vi "N-216 Test Panel - DLL.vi"() -> ()   [LabVIEW 2016]
uses:
  PI GCS2 DLL/PI_GCS2_DLL_x64.dll
panel:
  in  "Num of Axes":i32=1
  out "Axes Names":string
  in  "Query All Connected":bool
  out "MVR Success":u8
  in  "Move Relative":dbl
  out "Set VEL Success":u8
  in  "Set Velocity (µm/s)":dbl
  out "Velocities":dbl[](array[numeric])
  in  "Get Velocity (um/sec)":bool
  out "Halt Cmd Success":u8
  in  "Halt":bool
  out "ONT? Success":u8
  out "ONT?":u8[](array[numeric])
  in  "Check On Target":bool
  out "MOV Cmd Success":u8
  in  "Move to Position (µm)":dbl
  out "Referencing":bool
  out "Reference Position":dbl[](array[numeric])
  in  "Perform REF":bool
  out "FRF?":u8[](array[numeric])
  out "FRF Success":u8
  in  "Check REF":bool
  out "SVO Return":u8
  in  "SVO":bool
  in  "Axis":string="1"
  in  "All Axis":bool=TRUE
  in  "Get SVO State":bool
  in  "Get Position":bool
  in  "Quit":bool
  out "Error Code":i32
  out "Servo States":u8[](array[numeric])
  out "Positions":dbl[](array[numeric])
  out "Device ID":i32
  out "PI USB Devices":string
  out "Number Connected":i32
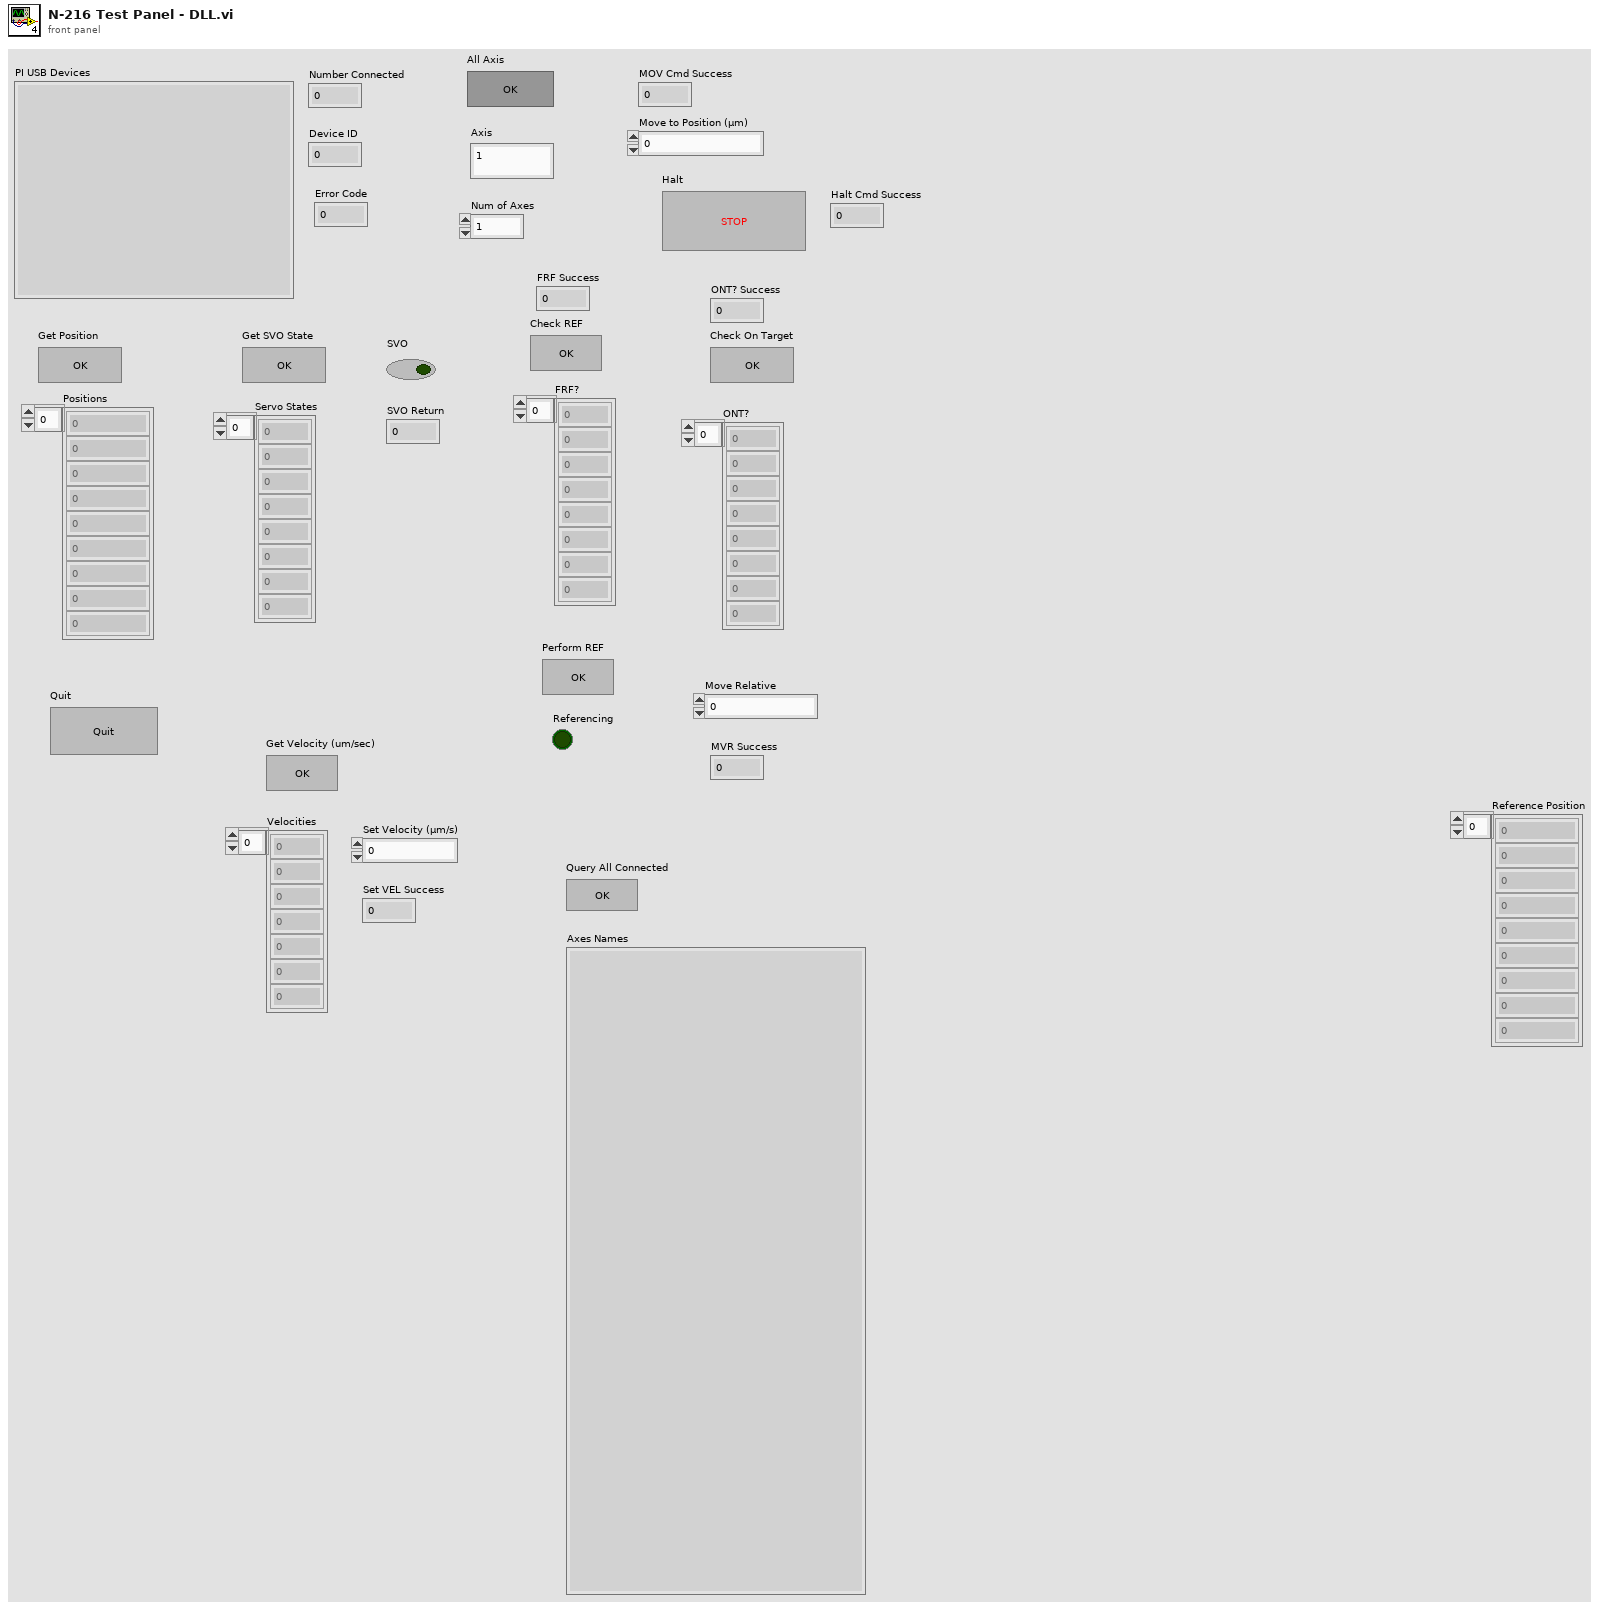
[diagram p1: front panel]
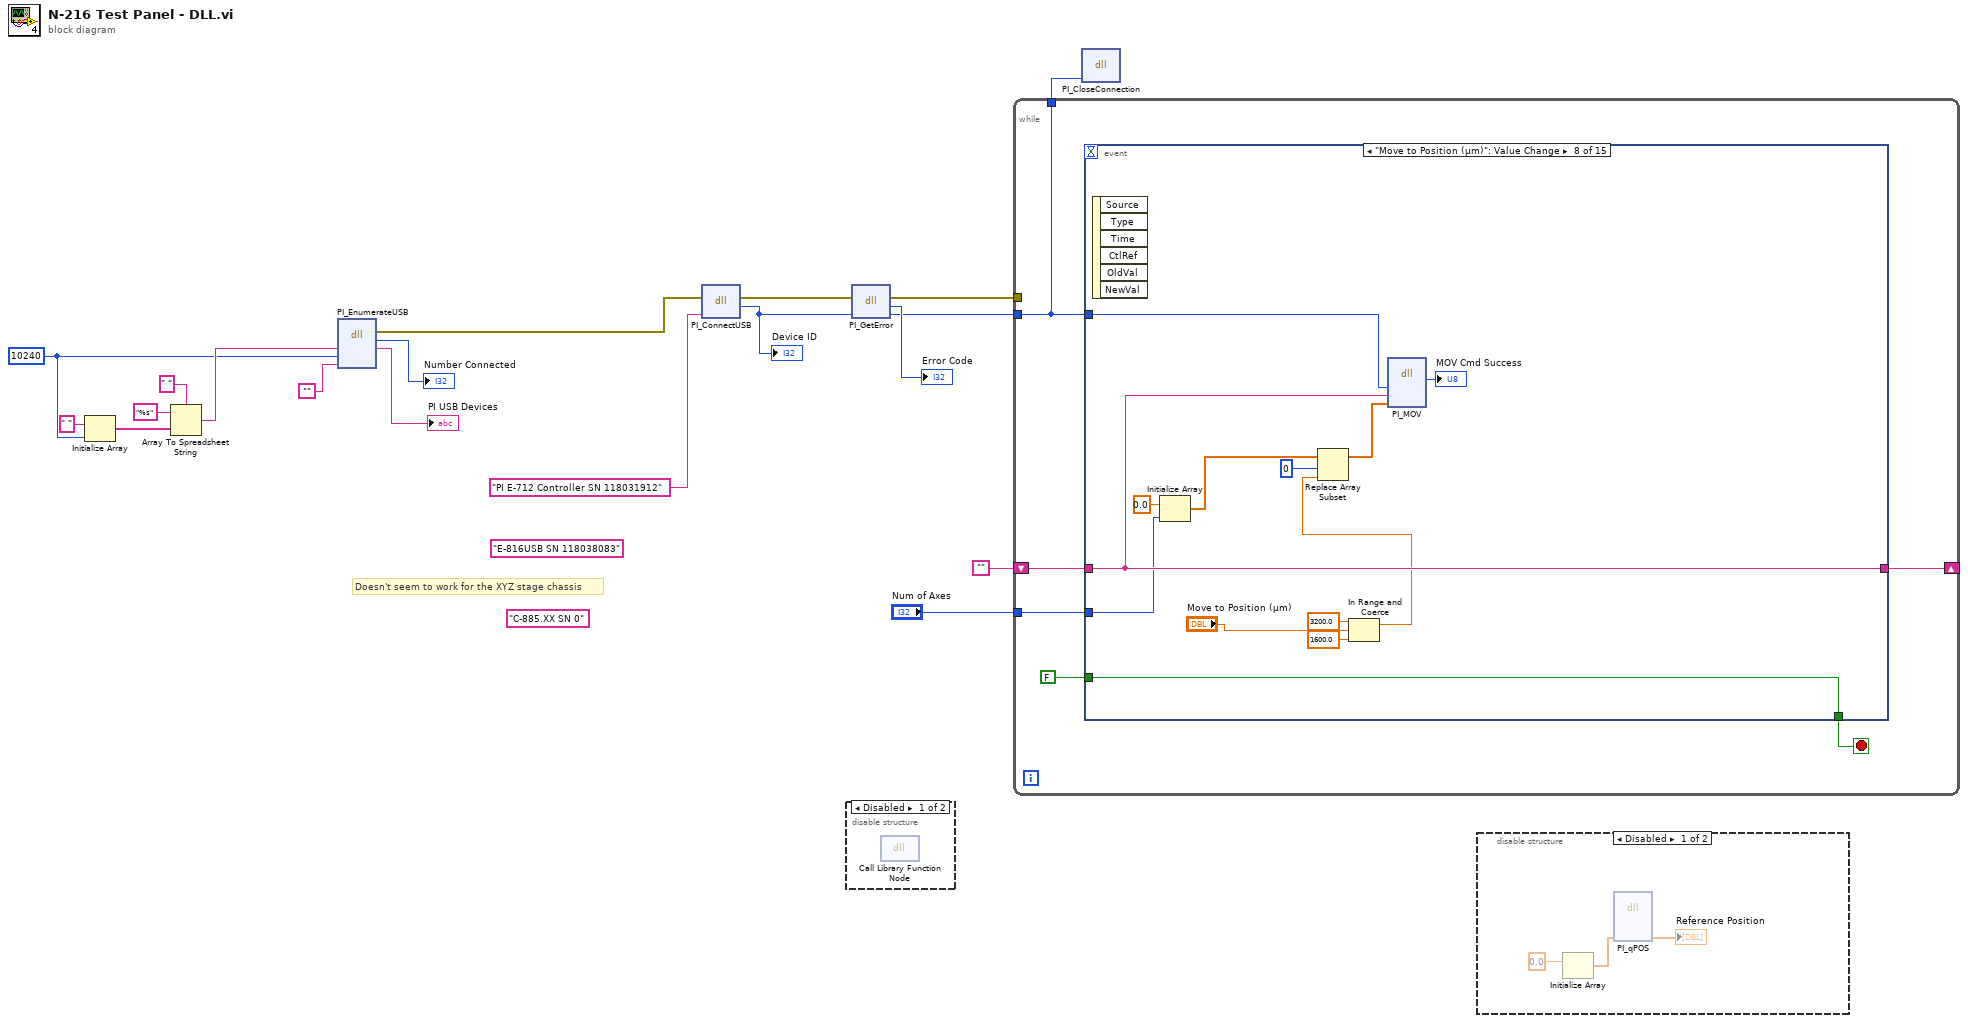
[diagram p0: block diagram]
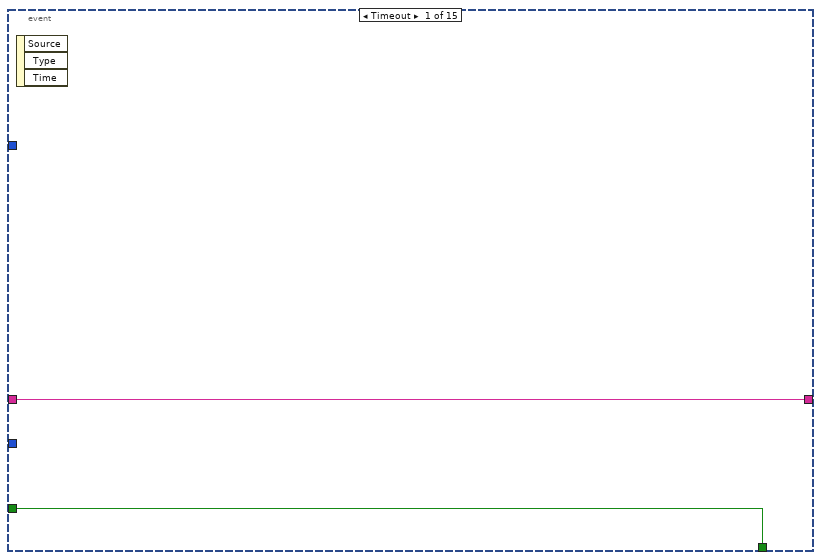
[diagram p3: hidden frame]
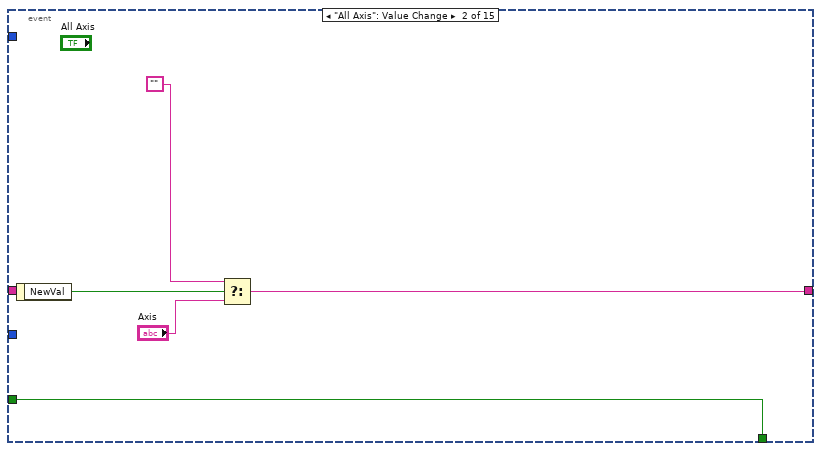
[diagram p4: hidden frame]
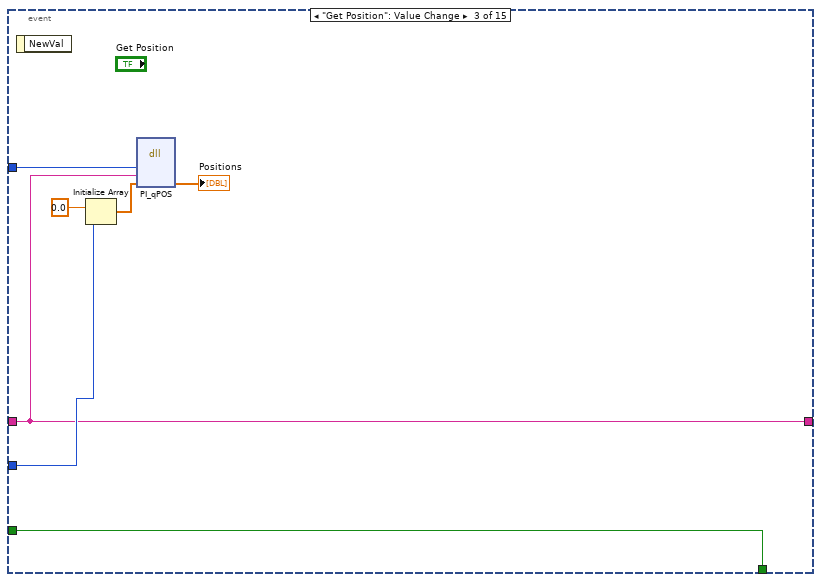
[diagram p5: hidden frame]
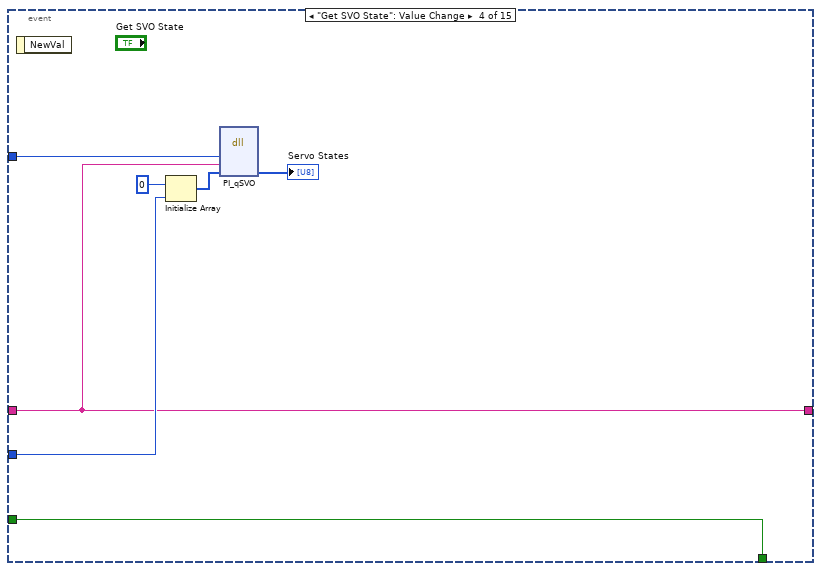
[diagram p6: hidden frame]
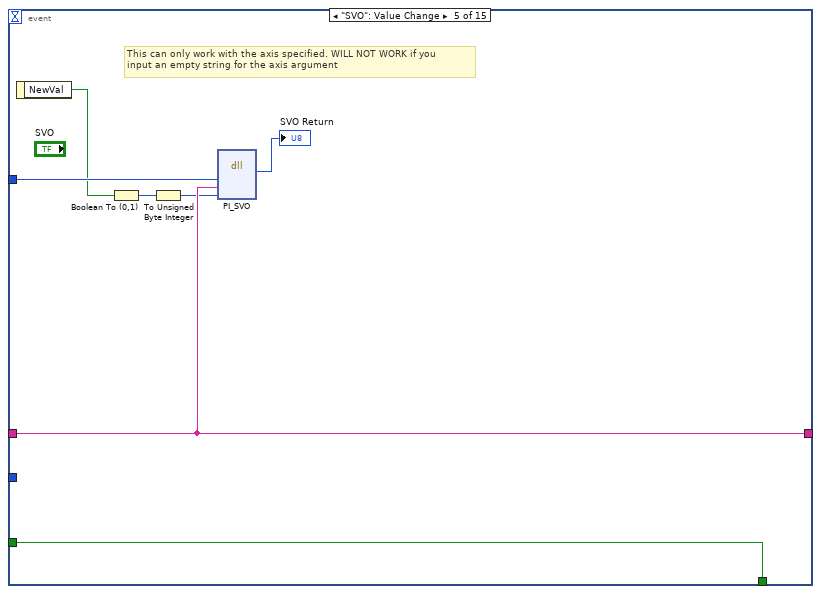
[diagram p7: hidden frame]
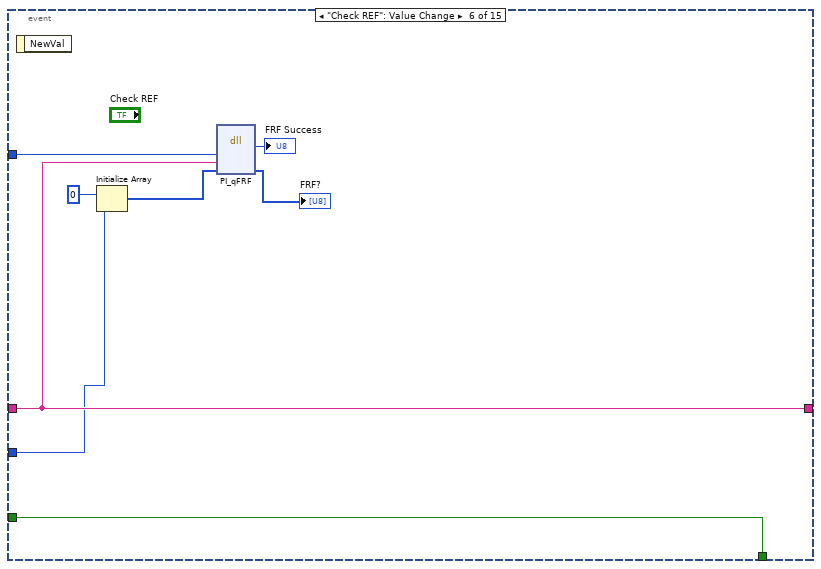
[diagram p8: hidden frame]
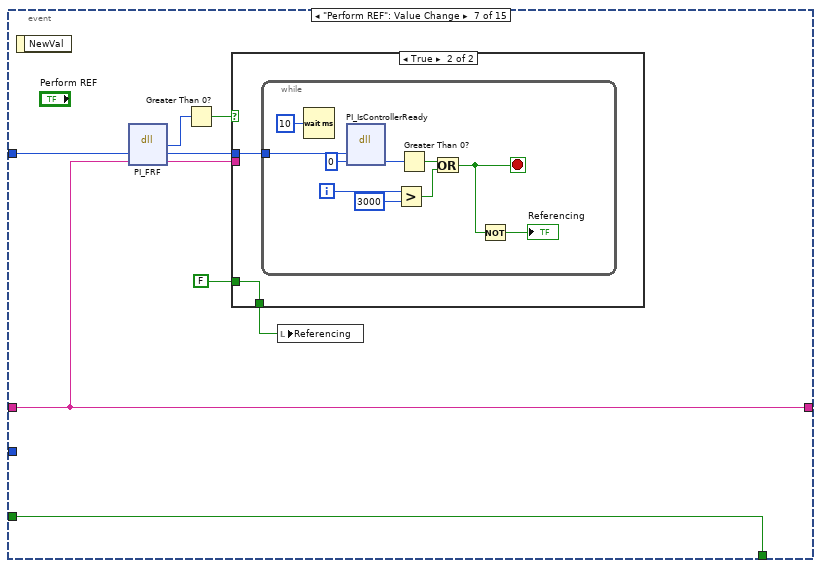
[diagram p9: hidden frame]
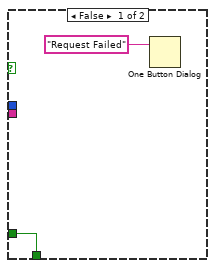
[diagram p10: hidden frame]
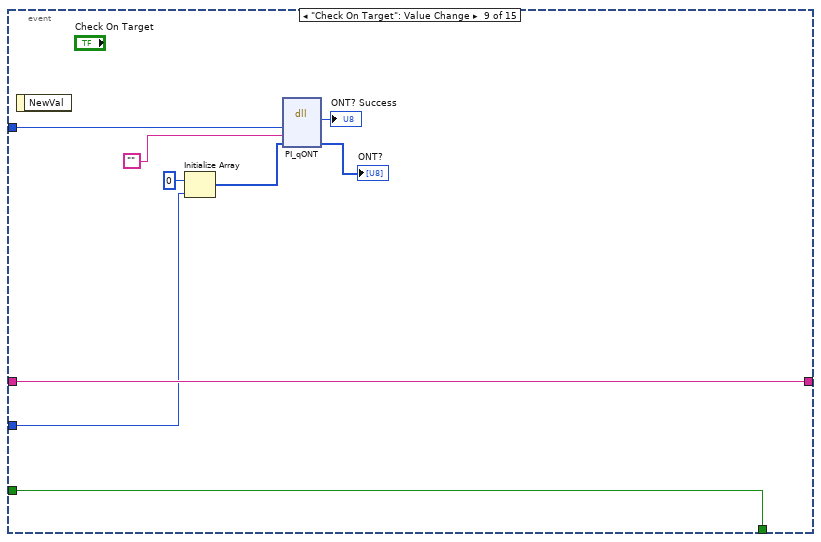
[diagram p11: hidden frame]
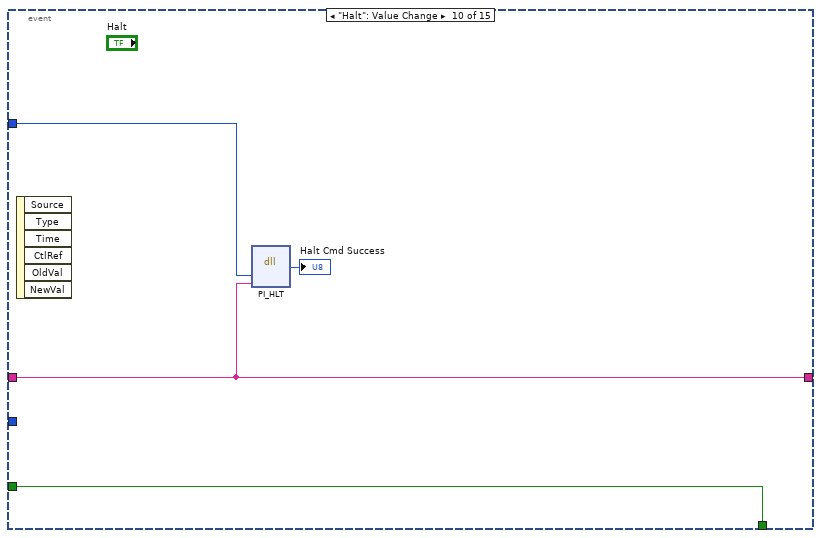
[diagram p12: hidden frame]
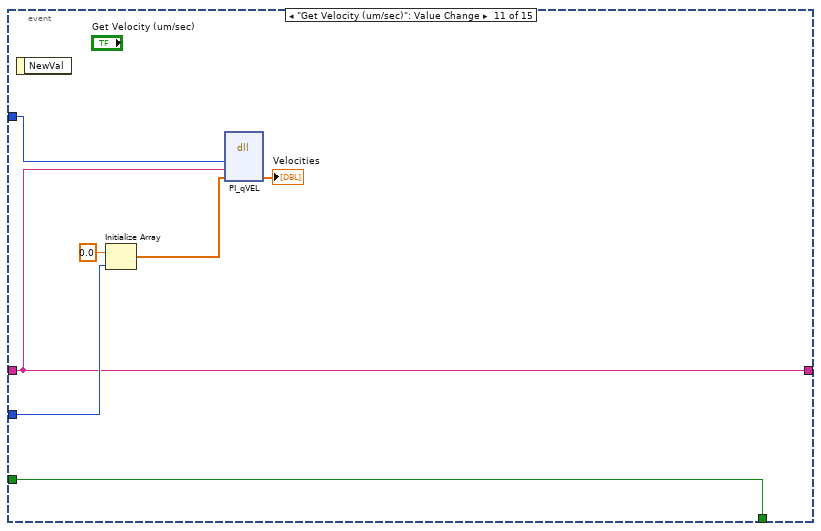
[diagram p13: hidden frame]
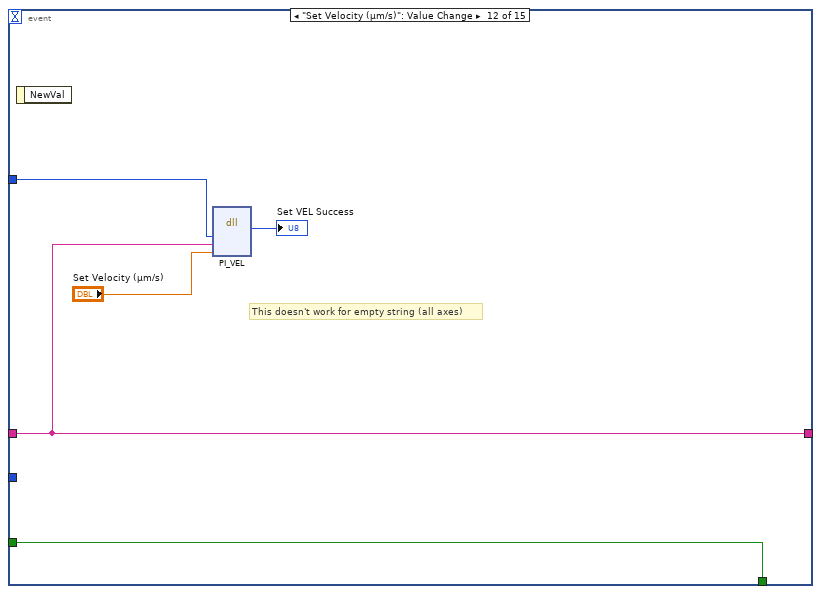
[diagram p14: hidden frame]
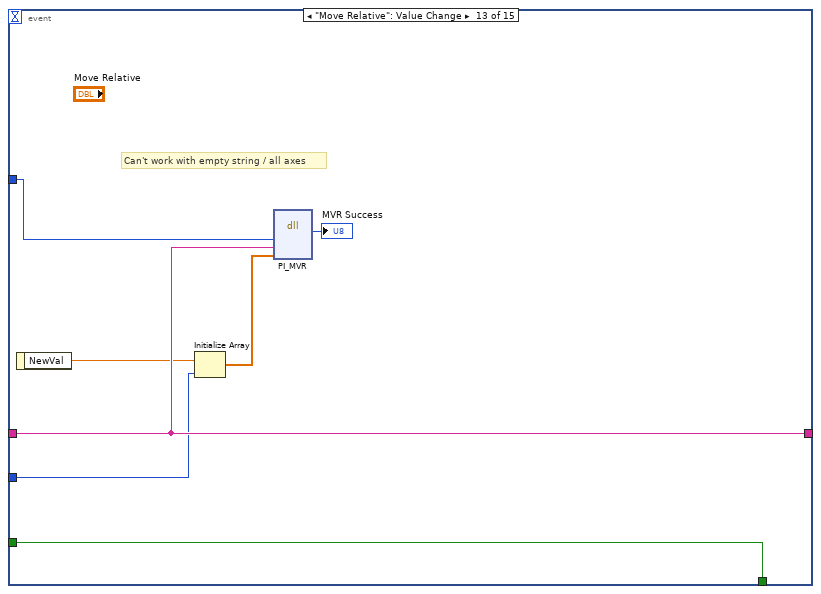
[diagram p15: hidden frame]
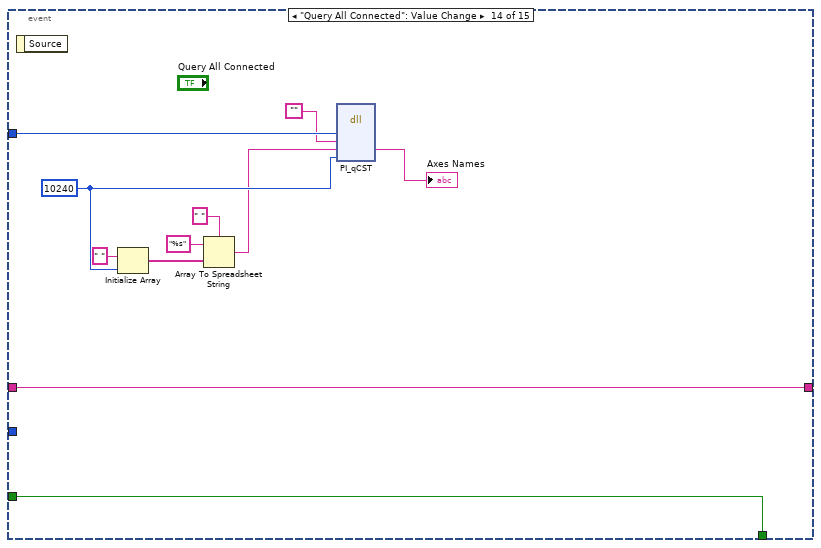
[diagram p16: hidden frame]
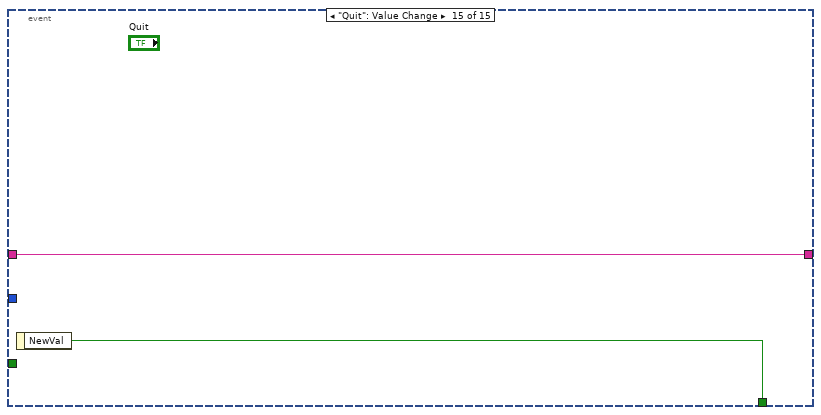
[diagram p17: hidden frame]
diagram:
  (unwired) "C-885.XX SN 0"
  (unwired) "E-816USB SN 118038083"
  w13 = 10240 ("dimension size")
  # "Doesn't seem to work for the XYZ stage chassis"
  n1 = Initialize Array(" ", w13) -> (w17:string[])
  n2 = Array To Spreadsheet String(delimiter (Tab)=" ", array=w17, 3:"%s" ("format string")) -> (spreadsheet string=w14:string)
  n3 = dll-call lib="C:/Users/George Sirinakis/Documents/Microscope-Control/Device Library/Stages/PI/PI GCS2 DLL/PI_GCS2_DLL_x64.dll" fn="PI_EnumerateUSB"("szBuffer"=w14, "iBufferSize"=w13, "szFilter"="") -> (error out=w10:errorcluster, "return type"=→"Number Connected":i32, "szBuffer"=→"PI USB Devices":string)  [unwired: 5 in, 1 out]
  n4 = dll-call lib="C:/Users/George Sirinakis/Documents/Microscope-Control/Device Library/Stages/PI/PI GCS2 DLL/PI_GCS2_DLL_x64.dll" fn="PI_ConnectUSB"(error in=w10, "szDescription"="PI E-712 Controller SN 118031912" ("delimiter (Tab)")) -> (error out=w9:errorcluster, "return type"=w8:i32)  [unwired: 3 in, 1 out]
  "Device ID" <- w8
  n5 = disable-structure shown="Disabled" {
    frame Disabled {
      n6 = dll-call lib="C:/Users/George Sirinakis/Documents/Microscope-Control/Device Library/Stages/PI/PI GCS2 DLL/PI_GCS2_DLL_x64.dll" fn="Call Library Function Node"() -> ()  [unwired: 4 in, 2 out]
    }
    frame Enabled {
    }
  }
  n7 = dll-call lib="C:/Users/George Sirinakis/Documents/Microscope-Control/Device Library/Stages/PI/PI GCS2 DLL/PI_GCS2_DLL_x64.dll" fn="PI_GetError"(error in=w9, "Device ID"=w8) -> (error out=w6:errorcluster, "Error Code"=→"Error Code":i32, "Device ID"=w5:i32)  [unwired: 2 in, 1 out]
  n8 = while {
    tunnel: w6 -> [_]
    tunnel: w5 -> [w20]
    shift-right: [w23] -> _
    shift-left: "" -> [w22]
    tunnel: "Num of Axes" -> [w21]
    tunnel: [w20] -> w2
    stop <- w25 stop-if-true
    n9 = event shown="[7] \"Move to Position (µm)\": Value Change" {
      selector: _ -> [_ _ _ _ _ _ _ _ _ _ _ _ _ _ _]
      dyn-events: _ -> [_ _ _ _ _ _ _ _ _ _ _ _ _ _ _]
      timeout: _ -> [_ _ _ _ _ _ _ _ _ _ _ _ _ _ _]
      tunnel: [w27 w32 w39 w40 w53 w61 w70 w94 w106 w107 w111 w122 w129 w130 w142] -> w25
      tunnel: FALSE -> [w27 w32 w39 w40 w53 w61 w70 w94 w106 w107 w111 w122 w129 w130 _]
      tunnel: [w26 w28 w33 w41 w50 w59 w67 w95 w104 w110 w112 w120 w128 w131 w141] -> w23
      tunnel: w20 -> [_ _ w35 w42 w52 w60 w69 w97 w105 w109 w117 w121 w127 w134 _]
      tunnel: w22 -> [w26 _ w33 w41 w50 w59 w67 w95 w104 w110 w112 w120 w128 w131 w141]
      tunnel: w21 -> [_ _ w34 w43 _ w57 _ w92 w103 _ w116 _ w124 _ _]
      event Timeout {
        n10 = event-data() -> ()  [unwired: 1 in, 3 out]
      }
      event "All Axis": Value Change {
        n11 = event-data() -> ("NewVal"=w31:bool)  [unwired: 1 in]
        n12 = Select(t="", s=w31, f="Axis") -> (s? t:f=w28:string)
      }
      event "Get Position": Value Change {
        n13 = event-data() -> ()  [unwired: 1 in, 1 out]
        n14 = Initialize Array(0.0 ("element"), w34) -> (w37:dbl[])
        n15 = dll-call lib="C:/Users/George Sirinakis/Documents/Microscope-Control/Device Library/Stages/PI/PI GCS2 DLL/PI_GCS2_DLL_x64.dll" fn="PI_qPOS"("ID"=w35, "szAxes"=w33, "pdValueArray"=w37) -> ("pdValueArray"=→"Positions":dbl[])  [unwired: 6 in, 2 out]
      }
      event "Get SVO State": Value Change {
        n16 = event-data() -> ()  [unwired: 1 in, 1 out]
        n17 = Initialize Array(u8 0 ("element"), w43) -> (w45:u8[])
        n18 = dll-call lib="C:/Users/George Sirinakis/Documents/Microscope-Control/Device Library/Stages/PI/PI GCS2 DLL/PI_GCS2_DLL_x64.dll" fn="PI_qSVO"("Device ID"=w42, "szAxes"=w41, "pdValueArray"=w45) -> ("pdValueArray"=→"Servo States":u8[])  [unwired: 6 in, 2 out]
      }
      event "SVO": Value Change {
        # "This can only work with the axis specified. WILL NOT WORK if you\ninput an empty string for the axis argument"
        n19 = event-data() -> ("NewVal"=w49:bool)  [unwired: 1 in]
        n20 = Boolean To (0,1)(Boolean=w49) -> (0, 1=w48:i16)
        n21 = To Unsigned Byte Integer(number=w48) -> (unsigned 8bit integer=w47:u8)
        n22 = dll-call lib="C:/Users/George Sirinakis/Documents/Microscope-Control/Device Library/Stages/PI/PI GCS2 DLL/PI_GCS2_DLL_x64.dll" fn="PI_SVO"("Device ID"=w52, "szAxes"=w50, "pdValueArray"=w47) -> ("Bool"=→"SVO Return":u8)  [unwired: 6 in, 2 out]
      }
      event "Check REF": Value Change {
        n23 = event-data() -> ()  [unwired: 1 in, 1 out]
        n24 = Initialize Array(u8 0 ("element"), w57) -> (w56:u8[])
        n25 = dll-call lib="C:/Users/George Sirinakis/Documents/Microscope-Control/Device Library/Stages/PI/PI GCS2 DLL/PI_GCS2_DLL_x64.dll" fn="PI_qFRF"("Device ID"=w60, "szAxes"=w59, "pdValueArray"=w56) -> ("Success"=→"FRF Success":u8, "pdValueArray"=→"FRF?":u8[])  [unwired: 5 in, 2 out]
      }
      event "Perform REF": Value Change {
        n26 = event-data() -> ()  [unwired: 1 in, 1 out]
        n27 = dll-call lib="C:/Users/George Sirinakis/Documents/Microscope-Control/Device Library/Stages/PI/PI GCS2 DLL/PI_GCS2_DLL_x64.dll" fn="PI_FRF"("Device ID"=w69, "szAxes"=w67) -> ("Success"=w68:u8, "Device ID"=w65:i32, "szAxes"=w64:string)  [unwired: 3 in, 2 out]
        n28 = Greater Than 0?(x=w68) -> (x > 0?=w66:bool)
        n29 = case shown="True" w66 {
          tunnel: w65 -> [_ w74]
          tunnel: w64 -> [_ _]
          tunnel: FALSE -> [w71 w73]
          tunnel: [w71 w73] -> w62
          frame False {
            n30 = One Button Dialog(message="Request Failed") -> ()  [unwired: 1 in, 1 out]
          }
          frame True {
            n31 = while {
              tunnel: w74 -> [w84]
              i -> [w82]
              stop <- w76 stop-if-true
              n32 = Wait (ms)(milliseconds to wait=u32 10) -> ()  [unwired: 1 out]
              n33 = dll-call lib="C:/Users/George Sirinakis/Documents/Microscope-Control/Device Library/Stages/PI/PI GCS2 DLL/PI_GCS2_DLL_x64.dll" fn="PI_IsControllerReady"("Device ID"=w84, "piControllerReady"=0) -> ("piControllerReady"=w79:i32)  [unwired: 5 in, 2 out]
              n34 = Greater?(x=w82, y=3000) -> (0:w77:bool)
              n35 = Greater Than 0?(x=w79) -> (x > 0?=w78:bool)
              n36 = Or(x=w78, y=w77) -> (x .or. y?=w76:bool)
              n37 = Not(x=w76) -> (.not. x?=→"Referencing":bool)
            }
          }
        }
        n38 = local write "Referencing"(w62) -> ()
      }
      event "Move to Position (µm)": Value Change {
        n39 = event-data() -> ()  [unwired: 1 in, 6 out]
        n40 = Initialize Array(0.0 ("element"), w92) -> (w91:dbl[])
        n41 = In Range and Coerce(upper limit=3200.0, x="Move to Position (µm)", lower limit=1600.0) -> (coerced(x)=w85:dbl)  [unwired: 1 out]
        n42 = Replace Array Subset(array=w91, new element=w85, index=0) -> (w89:dbl[])
        n43 = dll-call lib="C:/Users/George Sirinakis/Documents/Microscope-Control/Device Library/Stages/PI/PI GCS2 DLL/PI_GCS2_DLL_x64.dll" fn="PI_MOV"("Device ID"=w97, "szAxes"=w95, "pdValueArray"=w89) -> ("Success"=→"MOV Cmd Success":u8)  [unwired: 6 in, 2 out]
      }
      event "Check On Target": Value Change {
        n44 = event-data() -> ()  [unwired: 1 in, 1 out]
        n45 = Initialize Array(u8 0 ("element"), w103) -> (w101:u8[])
        n46 = dll-call lib="C:/Users/George Sirinakis/Documents/Microscope-Control/Device Library/Stages/PI/PI GCS2 DLL/PI_GCS2_DLL_x64.dll" fn="PI_qONT"("Device ID"=w105, "szAxes"="", "pdValueArray"=w101) -> ("Success"=→"ONT? Success":u8, "pdValueArray"=→"ONT?":u8[])  [unwired: 5 in, 2 out]
      }
      event "Halt": Value Change {
        n47 = event-data() -> ()  [unwired: 1 in, 6 out]
        n48 = dll-call lib="C:/Users/George Sirinakis/Documents/Microscope-Control/Device Library/Stages/PI/PI GCS2 DLL/PI_GCS2_DLL_x64.dll" fn="PI_HLT"("Device ID"=w109, "szAxes"=w110) -> ("Success"=→"Halt Cmd Success":u8)  [unwired: 5 in, 2 out]
      }
      event "Get Velocity (um/sec)": Value Change {
        n49 = event-data() -> ()  [unwired: 1 in, 1 out]
        n50 = Initialize Array(0.0 ("element"), w116) -> (w114:dbl[])
        n51 = dll-call lib="C:/Users/George Sirinakis/Documents/Microscope-Control/Device Library/Stages/PI/PI GCS2 DLL/PI_GCS2_DLL_x64.dll" fn="PI_qVEL"("Device ID"=w117, "szAxes"=w112, "pdValueArray"=w114) -> ("pdValueArray"=→"Velocities":dbl[])  [unwired: 6 in, 2 out]
      }
      event "Set Velocity (µm/s)": Value Change {
        # "This doesn't work for empty string (all axes)"
        n52 = event-data() -> ()  [unwired: 1 in, 1 out]
        n53 = dll-call lib="C:/Users/George Sirinakis/Documents/Microscope-Control/Device Library/Stages/PI/PI GCS2 DLL/PI_GCS2_DLL_x64.dll" fn="PI_VEL"("Device ID"=w121, "szAxes"=w120, "pdValueArray"="Set Velocity (µm/s)") -> ("Success"=→"Set VEL Success":u8)  [unwired: 6 in, 2 out]
      }
      event "Move Relative": Value Change {
        # "Can't work with empty string / all axes"
        n54 = event-data() -> ("NewVal"=w125:dbl)  [unwired: 1 in]
        n55 = Initialize Array(w125, w124) -> (w123:dbl[])
        n56 = dll-call lib="C:/Users/George Sirinakis/Documents/Microscope-Control/Device Library/Stages/PI/PI GCS2 DLL/PI_GCS2_DLL_x64.dll" fn="PI_MVR"("Device ID"=w127, "szAxes"=w128, "pdValueArray"=w123) -> ("Success"=→"MVR Success":u8)  [unwired: 6 in, 2 out]
      }
      event "Query All Connected": Value Change {
        w136 = 10240 ("dimension size")
        n57 = event-data() -> ()  [unwired: 1 in, 1 out]
        n58 = Initialize Array(" ", w136) -> (w139:string[])
        n59 = Array To Spreadsheet String(delimiter (Tab)=" ", array=w139, 3:"%s" ("format string")) -> (spreadsheet string=w135:string)
        n60 = dll-call lib="C:/Users/George Sirinakis/Documents/Microscope-Control/Device Library/Stages/PI/PI GCS2 DLL/PI_GCS2_DLL_x64.dll" fn="PI_qCST"("Device ID"=w134, "szAxes"="", "szNames"=w135, "iBufferSize"=w136) -> ("szNames"=→"Axes Names":string)  [unwired: 7 in, 2 out]
      }
      event "Quit": Value Change {
        n61 = event-data() -> ("NewVal"=w142:bool)  [unwired: 1 in]
      }
    }
  }
  n62 = dll-call lib="C:/Users/George Sirinakis/Documents/Microscope-Control/Device Library/Stages/PI/PI GCS2 DLL/PI_GCS2_DLL_x64.dll" fn="PI_CloseConnection"("ID"=w2) -> ()  [unwired: 5 in, 2 out]
  n63 = disable-structure shown="Disabled" {
    frame Disabled {
      n64 = Initialize Array(0.0 ("element")) -> (w144:dbl[])  [unwired: 1 in]
      n65 = dll-call lib="C:/Users/George Sirinakis/Documents/Microscope-Control/Device Library/Stages/PI/PI GCS2 DLL/PI_GCS2_DLL_x64.dll" fn="PI_qPOS"("pdValueArray"=w144) -> ("pdValueArray"=→"Reference Position":dbl[])  [unwired: 8 in, 2 out]
    }
    frame Enabled {
    }
  }
